vi "test_UDP_UDP Write.vi"(8 "error in (no error)":errorcluster, 11 "TestCase in":refnum<class "Ethernet Protocol Tests.lvclass">) -> (0 "error out":errorcluster, 3 "TestCase out":refnum<class "Ethernet Protocol Tests.lvclass">)   [LabVIEW 2019, in "Ethernet Protocol Tests.lvclass"]
uses:
  Ethernet Protocol Tests.lvclass
  UDP/UDP.lvclass
  D:/GitRepository/niveristand-instrument-addon-classes/Source/Protocols/Protocol Parent/Protocol Parent.lvclass
  Listener/Listener.lvclass
  Listener/ListenerClassControls/Operation.ctl
  UDP/UDP.lvclass/UDP.ctl
  UDP/Data Access/Write Local IP Address.vi
  UDP/Data Access/Write Target IP Address.vi
  UDP/Data Access/Write Local Port.vi
  UDP/Data Access/Write Target Port.vi
  <vilib>/addons/_JKI Toolkits/VI Tester/TestCase.llb/TestCase.lvclass
  C:/Program Files (x86)/National Instruments/LabVIEW 2019/vi.lib/addons/_JKI Toolkits/VI Tester/TestCase.llb/TestCase.lvclass
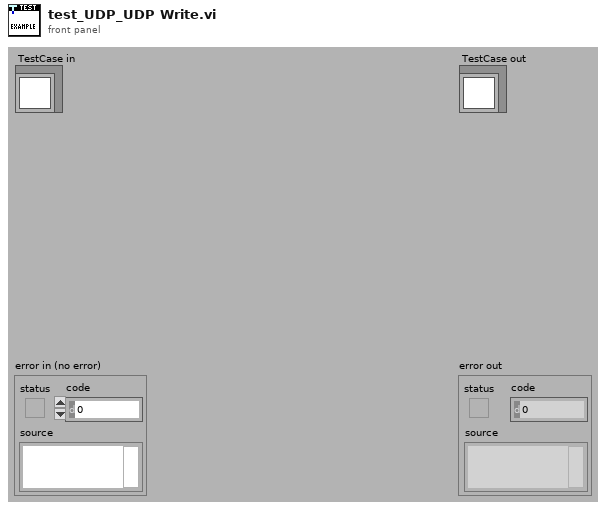
[diagram p1: front panel]
types:
  T1 = typedef "Listener.lvclass/Operation.ctl" = enum16{"Read", "Write"}
  T2 = typedef "Listener.lvclass/UDP Data Structure.ctl" = cluster{"UDP connection ID":refnum<k16>, "Local Address":string, "Local Port":u16, "Target IP Address":string, "Target Port":u16, "Data":string}
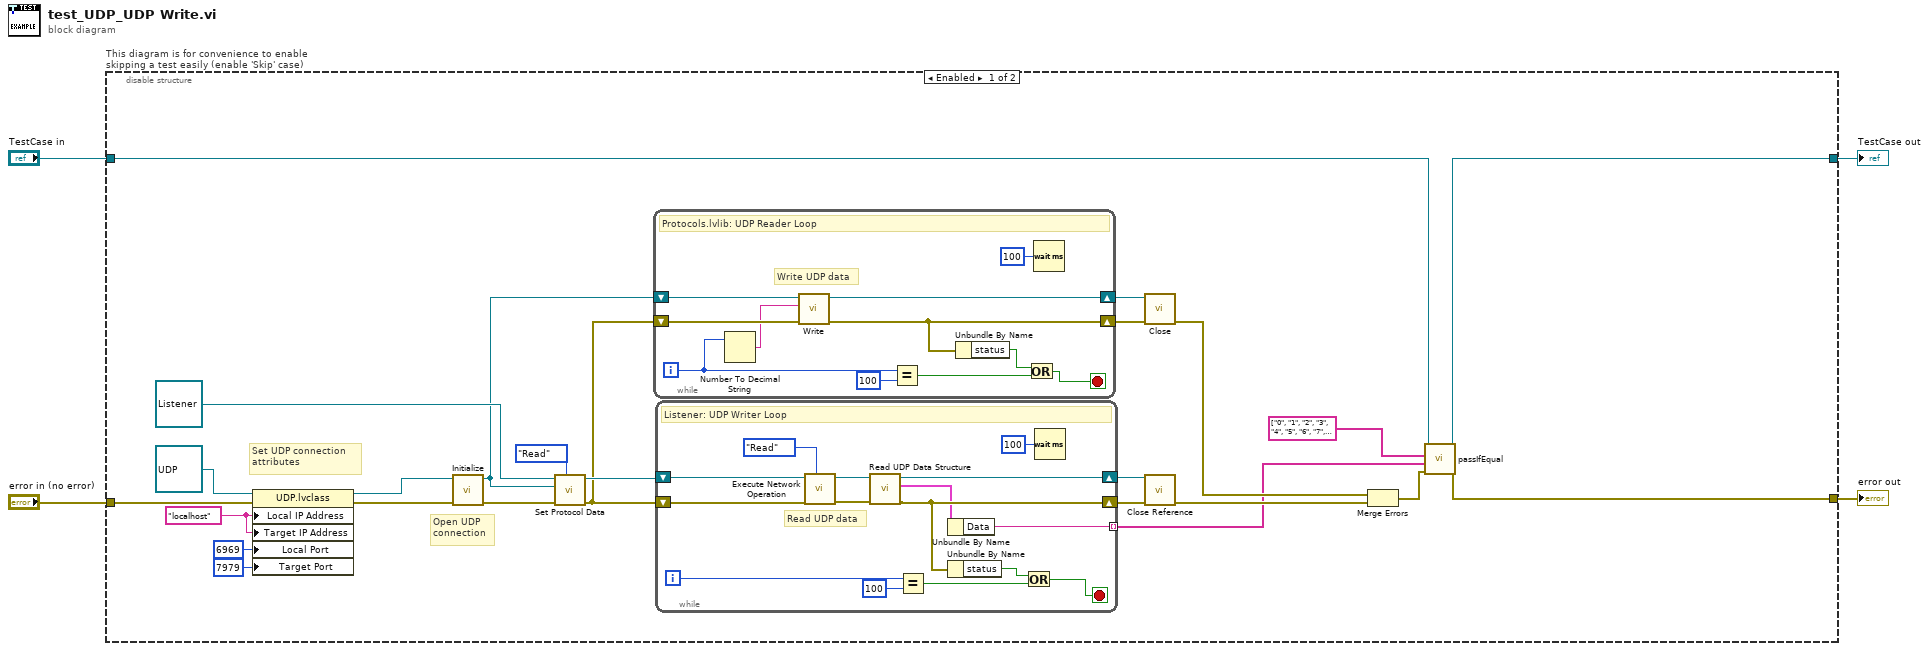
[diagram p0: block diagram]
diagram:
  n1 = disable-structure "This diagram is for convenience to enable skipping a test easily (enable 'Skip' case)" shown="Enabled" {
    disable-tunnel: "TestCase in" -> [w29 w59]
    disable-tunnel: [w28 w57] -> w1
    disable-tunnel: [w27 w58] -> w3
    disable-tunnel: "error in (no error)" -> [w25 w56]
    frame Enabled {
      w15 = "localhost" ("Local IP Address")
      # "Open UDP \nconnection"
      # "Set UDP connection \nattributes"
      n2 = property class="UDP.lvclass"(reference=refnum<class "UDP.lvclass"> refnum ("Protocols.lvlib:UDP.lvclass"), error in=w25, "Local IP Address"=w15, "Target IP Address"=w15, "Local Port"=u16 6969, "Target Port"=u16 7979) -> (reference out=w24:refnum<class "UDP.lvclass">, error out=w23:errorcluster)
      n3 = call-dynamic "Initialize.vi"("error in (no error)"=w23, "UDP in"=w24) -> ("error out"=w22:errorcluster, "UDP out"=w19:refnum<class "UDP.lvclass">)  [unwired: 8 in]
      n4 = call "Set Protocol Data.vi"("Operation"=Operation."Read", "error in (no error)"=w22, "Protocols.lvlib:Protocol Parent.lvclass"=w19, "Listener In.lvclass"=refnum<class "Listener.lvclass"> refnum ("Listener.lvclass")) -> ("error out"=w18:errorcluster, "Listener Out.lvclass"=w20:refnum<class "Listener.lvclass">)  [unwired: 6 in]
      n5 = while {
        shift-right: [w45] -> w11
        shift-left: w18 -> [w51]
        shift-right: [w49] -> w10
        shift-left: w19 -> [w50]
        i -> [w48]
        stop <- w52 stop-if-true
        # "Write UDP data"
        # "Protocols.lvlib: UDP Reader Loop"
        n6 = Number To Decimal String(number=w48) -> (decimal integer string=w47:string)  [unwired: 1 in]
        n7 = call-dynamic "Write.vi"("error in (no error)"=w51, "String"=w47, "UDP in"=w50) -> ("error out"=w45:errorcluster, "UDP out"=w49:refnum<class "UDP.lvclass">)  [unwired: 7 in]
        n8 = Equal?(x=w48, y=100) -> (x = y?=w53:bool)
        n9 = Unbundle By Name(w45) -> ("status"=w46:bool)
        n10 = Or(x=w46, y=w53) -> (x .or. y?=w52:bool)
        n11 = Wait (ms)(milliseconds to wait=u32 100) -> ()  [unwired: 1 out]
      }
      n12 = while {
        shift-right: [w32] -> w7
        shift-left: w20 -> [w42]
        shift-right: [w33] -> w8
        shift-left: w18 -> [w44]
        tunnel: [w30] -> w5 mode=indexing
        i -> [w36]
        stop <- w37 stop-if-true
        # "Read UDP data"
        # "Listener: UDP Writer Loop"
        n13 = call "Execute Network Operation.vi"("Operation"=Operation."Read", "error in (no error)"=w44, "Listener In.lvclass"=w42) -> ("error out"=w35:errorcluster, "Listener Out.lvclass"=w34:refnum<class "Listener.lvclass">)  [unwired: 7 in]
        n14 = call-dynamic "Read UDP Data Structure.vi"("error in (no error)"=w35, "Listener in"=w34) -> ("error out"=w33:errorcluster, "UDP Data Structure"=w31:T2, "Listener out"=w32:refnum<class "Listener.lvclass">)  [unwired: 7 in]
        n15 = Equal?(x=w36, y=100) -> (x = y?=w39:bool)
        n16 = Unbundle By Name(w31) -> ("Data"=w30:string)
        n17 = Unbundle By Name(w33) -> ("status"=w38:bool)
        n18 = Or(x=w38, y=w39) -> (x .or. y?=w37:bool)
        n19 = Wait (ms)(milliseconds to wait=u32 100) -> ()  [unwired: 1 out]
      }
      n20 = call-dynamic "Close.vi"("error in (no error)"=w11, "UDP in"=w10) -> ("error out"=w9:errorcluster)  [unwired: 8 in, 1 out]
      n21 = call "Close Reference.vi"("error in (no error)"=w8, "Listener In.lvclass"=w7) -> ("error out"=w6:errorcluster)  [unwired: 9 in]
      n22 = Merge Errors(w9, w6) -> (w17:errorcluster)
      n23 = call-dynamic "passIfEqual.vi"("error in (no error)"=w17, "y"=w5, "x"=string[] ["0", "1", "2", "3", "4", "5", "6", "7", "8", "9", "10", "11", "12", "13", "14", "15", "16", "17", "18", "19", "20", "21", "22", "23", "24", "25", "26", "27", "28", "29", "30", "31", "32", "33", "34", "35", "36", "37", "38", "39", "40", "41", "42", "43", "44", "45", "46", "47", "48", "49", "50", "51", "52", "53", "54", "55", "56", "57", "58", "59", "60", "61", "62", "63", "64", "65", "66", "67", "68", "69", "70", "71", "72", "73", "74", "75", "76", "77", "78", "79", "80", "81", "82", "83", "84", "85", "86", "87", "88", "89", "90", "91", "92", "93", "94", "95", "96", "97", "98", "99", "100"] ("Array"), "TestCase in"=w29) -> ("error out"=w27:errorcluster, "TestCase out"=w28:refnum<class "Ethernet Protocol Tests.lvclass">)  [unwired: 6 in]
    }
    frame Disabled {
      # "skip test result while test is under development"
      n24 = call <vilib>:"skip.vi"("error in (no error)"=w56, "TestCase in"=w59) -> ("error out"=w58:errorcluster, "TestCase out"=w57:refnum<class "Ethernet Protocol Tests.lvclass">)  [unwired: 8 in]
    }
  }
  "error out" <- w3
  "TestCase out" <- w1
